vi "Remove_Tags.vi"(8 "error in (no error)":errorcluster, 11 "Input String":string) -> (0 "error out":errorcluster, 3 "Output String":string)   [LabVIEW 2018, in "MerriamWebsterJSON.lvlib"]
uses:
  MerriamWebsterJSON.lvlib
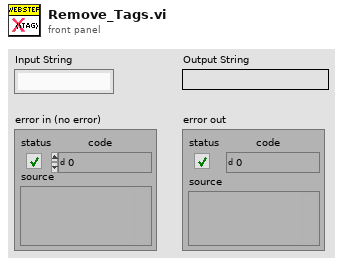
[diagram p1: front panel]
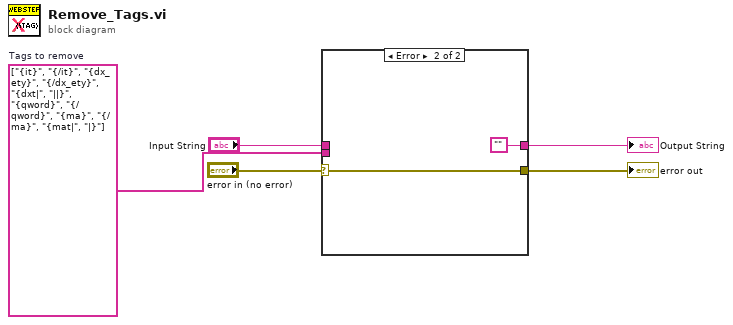
[diagram p0: block diagram]
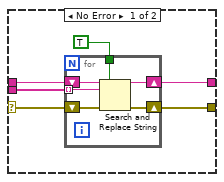
[diagram p2: hidden frame]
diagram:
  w5 = string[] ["{it}", "{/it}", "{dx_ety}", "{/dx_ety}", "{dxt|", "||}", "{qword}", "{/qword}", "{ma}", "{/ma}", "{mat|", "|}"]  # Tags to remove
  n1 = case shown="Error" "error in (no error)" {
    selector: "error in (no error)" -> [w7 w19]
    tunnel: w5 -> [w11 _]
    tunnel: "Input String" -> [w9 _]
    tunnel: [w8 ""] -> w3
    tunnel: [w6 w19] -> w1
    frame No Error {
      n2 = for {
        tunnel: w11 -> [w16] mode=indexing
        tunnel: TRUE ("replace all? (F)") -> [w17]
        shift-right: [w14] -> w8
        shift-left: w9 -> [w15]
        shift-right: [w12] -> w6
        shift-left: w7 -> [w13]
        n3 = Search and Replace String(replace all?=w17, input string=w15, search string=w16, error in=w13) -> (result string=w14:string, error out=w12:errorcluster)  [unwired: 4 in, 2 out]
      }
    }
    frame Error {
    }
  }
  "error out" <- w1
  "Output String" <- w3
